vi "WriteReadDescriptionToFolder.vi"(4 "F: Read/ T: Write (default)":bool=TRUE, 5 "error in":errorcluster, 6 "File name (default: Description.txt)":string="Description.txt", 7 "Description for folder in":string, 8 "Folder path":path) -> (0 "error out":errorcluster, 1 "Description exists?":bool, 2 "Description for folder out":string, 3 "Description File path":path)   [LabVIEW 2020, in "Initialization.lvlib" / "FileManagement.lvlib"]
uses:
  FileManagement.lvlib
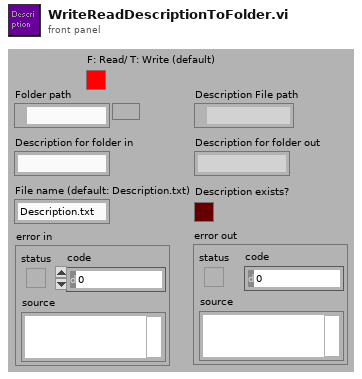
[diagram p1: front panel]
types:
  T1 = enum16{"open", "replace", "create", "open or create", "replace or create", "replace or create with confirmation"}
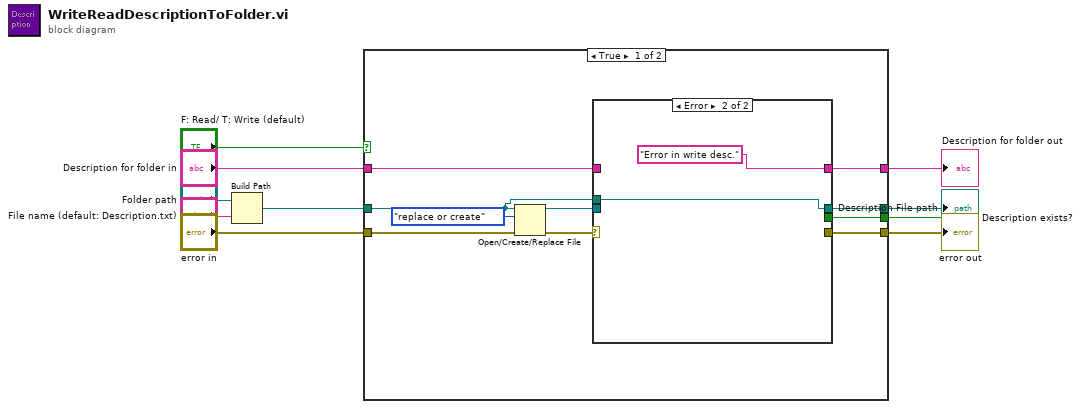
[diagram p0: block diagram]
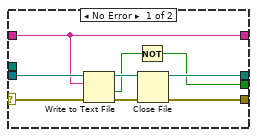
[diagram p2: hidden frame]
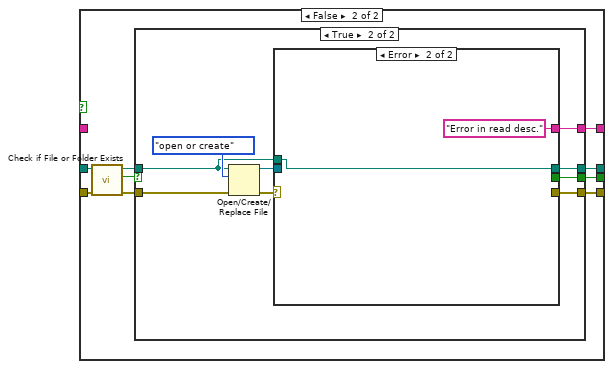
[diagram p3: hidden frame]
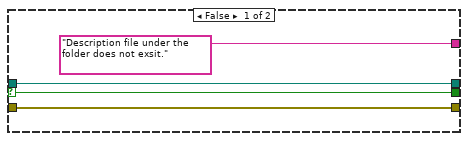
[diagram p4: hidden frame]
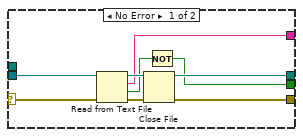
[diagram p5: hidden frame]
diagram:
  n1 = Build Path(base path="Folder path", name or relative path="File name (default: Description.txt)") -> (appended path=w9:path)
  n2 = case shown="True" "F: Read/ T: Write (default)" {
    tunnel: w9 -> [w12 w38]
    tunnel: "Description for folder in" -> [w16 _]
    tunnel: "error in" -> [w18 w37]
    tunnel: [w17 w40] -> w6
    tunnel: [w11 w33] -> w3
    tunnel: [w15 w39] -> w2
    tunnel: [w14 w32] -> w1
    frame True {
      n3 = Open/Create/Replace File(file path (use dialog)=w12, error in=w18, operation (0:open)=T1."replace or create") -> (refnum out=w19:refnum<file>, error out=w13:errorcluster)  [unwired: 3 in, 1 out]
      n4 = case shown="Error" w13 {
        selector: w13 -> [w22 _]
        tunnel: w19 -> [w29 _]
        tunnel: [w26 _] -> w17
        tunnel: w16 -> [w21 _]
        tunnel: [w25 w31] -> w15
        tunnel: [w24 _] -> w14
        tunnel: w12 -> [_ w31]
        tunnel: [w21 "Error in write desc."] -> w11
        frame No Error {
          n5 = Write to Text File(file (use dialog)=w29, text=w21, error in=w22) -> (refnum out=w27:refnum<file>, cancelled=w23:bool, error out=w28:errorcluster)  [unwired: 1 in]
          n6 = Not(x=w23) -> (.not. x?=w24:bool)
          n7 = Close File(refnum=w27, error in=w28) -> (path=w25:path, error out=w26:errorcluster)
        }
        frame Error {
        }
      }
    }
    frame False {
      n8 = call <vilib>:"Check if File or Folder Exists.vi"("error in (no error)"=w37, "path"=w38) -> ("error out"=w36:errorcluster, "file or folder exists?"=w34:bool, "dup path"=w35:path)  [unwired: 7 in]
      n9 = case shown="True" w34 {
        selector: w34 -> [w41 _]
        tunnel: [w43 w52] -> w40
        tunnel: [w44 w51] -> w39
        tunnel: w36 -> [w43 w50]
        tunnel: w35 -> [w44 w45]
        tunnel: ["Description file under the folder does not exsit." w48] -> w33
        tunnel: [w41 w47] -> w32
        frame False {
        }
        frame True {
          n10 = Open/Create/Replace File(file path (use dialog)=w45, error in=w50, operation (0:open)=T1."open or create") -> (refnum out=w53:refnum<file>, error out=w46:errorcluster)  [unwired: 3 in, 1 out]
          n11 = case shown="Error" w46 {
            selector: w46 -> [w54 _]
            tunnel: w53 -> [w62 _]
            tunnel: [w59 _] -> w52
            tunnel: [w58 w64] -> w51
            tunnel: [w57 "Error in read desc."] -> w48
            tunnel: [w55 _] -> w47
            tunnel: w45 -> [_ w64]
            frame No Error {
              n12 = Read from Text File(file (use dialog)=w62, error in=w54) -> (refnum out=w60:refnum<file>, text=w57:string, cancelled=w56:bool, error out=w61:errorcluster)  [unwired: 2 in]
              n13 = Close File(refnum=w60, error in=w61) -> (path=w58:path, error out=w59:errorcluster)
              n14 = Not(x=w56) -> (.not. x?=w55:bool)
            }
            frame Error {
            }
          }
        }
      }
    }
  }
  "error out" <- w6
  "Description for folder out" <- w3
  "Description File path" <- w2
  "Description exists?" <- w1
